vi "PathPlanner_PathPoint_New.vi"(8 "Rotation\nExists":bool, 9 "Constraints":T1, 10 "HolonomicRotation":T2={"VALUE"=0.0, "COS"=1.0, "SIN"=0.0} {"SIN" format="%13.4f"; "COS" format="%13.4f"; "VALUE" format="%13.4f"}, 11 "Position":T3 {"Y" format="%14.3f"; "X" format="%14.3f"}) -> (3 "PathPlannerPoint":T4={"Position"={"X"=0.0, "Y"=0.0}, "HolonomicRotation"={"VALUE"=0.0, "COS"=1.0, "SIN"=0.0}, "DistAlongPath"=0.0, "CurveRadius"=0.0, "MaxV"=9e+300, "Constraints"={"MaxVelocityMps;"=0.0, "MaxAccelerationMpsSq;"=0.0, "MaxAngularVelRadPsEc;"=0.0, "MaxAngularAccRadPSecSq"=0.0, "Exists"=FALSE}, "HolonomicRotationExists"=FALSE} {"HolonomicRotation"."SIN" format="%13.4f"; "HolonomicRotation"."COS" format="%13.4f"; "HolonomicRotation"."VALUE" format="%13.4f"; "Position"."Y" format="%14.3f"; "Position"."X" format="%14.3f"})   [LabVIEW 2019, in "PathPlanner24.lvlib"]
doc: "Create a path point\n \nInputs:\n -- position Position of the point\n -- holonomicRotation Rotation target at this point\n -- constraints The constraints at this point\n\nOutputs:\n -- PathPlannerPoint - cluster - point definition"
uses:
  PathPlanner24.lvlib
  TypeDef/PathPlannerPathPoint.ctl
  <vilib>/Rock Robotics/WPI/ThirdParty/JAS_Junk/TrajLib/TypeDef/TRANSLATION2D.ctl
  <vilib>/Rock Robotics/WPI/ThirdParty/JAS_Junk/TrajLib/TypeDef/ROTATION2D.ctl
  TypeDef/PathPlannerPathConstraints.ctl
  <vilib>/Rock Robotics/WPI/ThirdParty/JAS_Junk/TrajLib/Trajectory_Library.lvlib
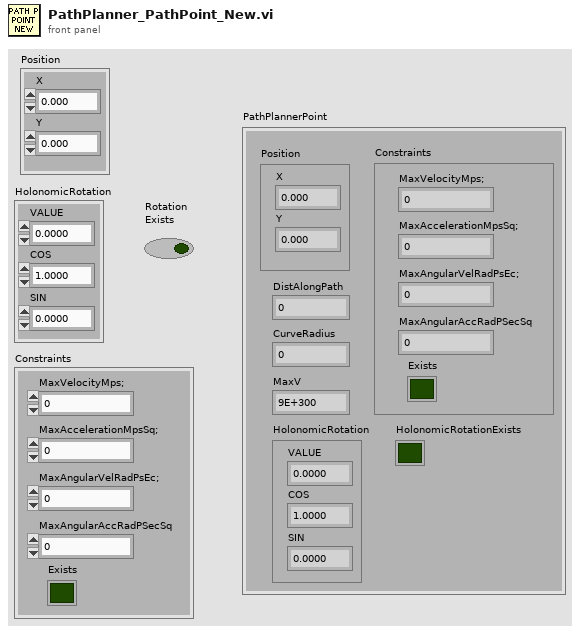
[diagram p1: front panel]
types:
  T1 = typedef "PathPlanner24.lvlib/PathPlannerPathConstraints.ctl" = cluster{"MaxVelocityMps;":dbl, "MaxAccelerationMpsSq;":dbl, "MaxAngularVelRadPsEc;":dbl, "MaxAngularAccRadPSecSq":dbl, "Exists":bool}
  T2 = typedef "Trajectory_Library.lvlib/ROTATION2D.ctl" = cluster{"VALUE":dbl, "COS":dbl, "SIN":dbl}
  T3 = typedef "Trajectory_Library.lvlib/TRANSLATION2D.ctl" = cluster{"X":dbl, "Y":dbl}
  T4 = typedef "PathPlanner24.lvlib/PathPlannerPathPoint.ctl" = cluster{"Position":T3, "HolonomicRotation":T2, "DistAlongPath":dbl, "CurveRadius":dbl, "MaxV":dbl, "Constraints":T1, "HolonomicRotationExists":bool}
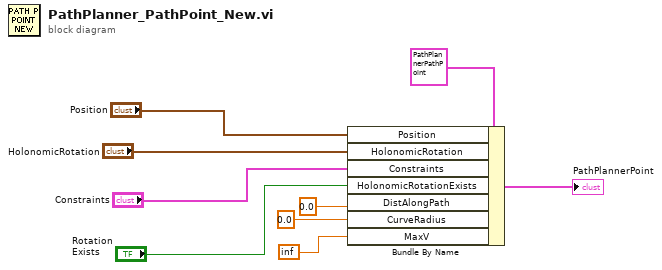
[diagram p0: block diagram]
diagram:
  n1 = Bundle By Name(cluster=T4 {"Position"={"X"=0.0, "Y"=0.0}, "HolonomicRotation"={"VALUE"=0.0, "COS"=1.0, "SIN"=0.0}, "DistAlongPath"=0.0, "CurveRadius"=0.0, "MaxV"=9e+300, "Constraints"={"MaxVelocityMps;"=0.0, "MaxAccelerationMpsSq;"=0.0, "MaxAngularVelRadPsEc;"=0.0, "MaxAngularAccRadPSecSq"=0.0, "Exists"=FALSE}, "HolonomicRotationExists"=FALSE} ("PathPlannerPoint"), "Position"="Position", "HolonomicRotation"="HolonomicRotation", "Constraints"="Constraints", "HolonomicRotationExists"="Rotation\nExists", "DistAlongPath"=0.0, "CurveRadius"=0.0, "MaxV"=inf) -> (→"PathPlannerPoint":T4)
